vi "user_config.vi"(11 "ClusterIn":T2={"Simulation?"=FALSE, "ChanConfigs"=[], "Test Config"={"HoleDiam"=1.4, "MeanLineDiam"=5.0, "IncF"=0.2, "ElastMod"=207.0, "PoissonMod"=0.3, "RosType"=enum."Tipo A", "Método de análise"=enum."Simplificado 2008", "Pfinal"=0.3, "AStop"=TRUE}, "Directory"=path "", "TestName"="", "RawFile"=refnum, "InfoFile"=refnum, "DataFile"=refnum, "task"="", "qRecord"=refnum, "qProcess"=refnum, "feed"=enum."Manual"} {"ChanConfigs"."GF" min=0.1 max=10.0; "ChanConfigs"."Canal" min=1 max=8}) -> (3 "ClusterOut":T2={"Simulation?"=FALSE, "ChanConfigs"=[], "Test Config"={"HoleDiam"=1.4, "MeanLineDiam"=5.0, "IncF"=0.2, "ElastMod"=207.0, "PoissonMod"=0.3, "RosType"=enum."Tipo A", "Método de análise"=enum."Simplificado 2008", "Pfinal"=0.3, "AStop"=TRUE}, "Directory"=path "", "TestName"="", "RawFile"=refnum, "InfoFile"=refnum, "DataFile"=refnum, "task"="", "qRecord"=refnum, "qProcess"=refnum, "feed"=enum."Manual"} {"ChanConfigs"."GF" min=0.1 max=10.0; "ChanConfigs"."Canal" min=1 max=8})   [LabVIEW 2016]
uses:
  Channel_config.ctl
  MainFGV/cluster_main_FGV.ctl
  test_config.ctl
  feedType.ctl
panel:
  in  "feed":T1 caption="Tipo de avanço"
  in  "ChanConfig":T3[](array[typedef])=[{"Canal"=1, "GF"=2.0, "SC"=FALSE}, {"Canal"=2, "GF"=2.0, "SC"=FALSE}, {"Canal"=3, "GF"=2.0, "SC"=FALSE}] {"GF" min=0.1 max=10.0; "Canal" min=1 max=8}
  in  "Parar auto.":bool=TRUE
  in  "Pf":dbl=1.0 caption="Profundidade final [mm]"
  in  "TR":enum16{"Tipo A", "Tipo B", "Tipo C"}(ring) caption="Tipo de roseta utilizada"
  in  "ni":dbl=0.3 caption="Módulo de Poisson"
  in  "E":dbl=207.0 caption="Módulo de elasticidade [GPa]"
  in  "IF":dbl=0.05 caption="Incremento de furação [mm]"
  in  "Dlm":dbl=5.13 caption="Diâmetro da linha média [mm]"
  in  "Df":dbl=1.4 caption="Diâmetro do furo [mm]"
  in  "Pronto":bool
  # "CONFIGURAÇÃO DO ENSAIO DE TENSÃO RESIDUAL"
  # "Informações essenciais para execução do ensaio"
  # "Sensor 1"
  # "Sensor 2"
  # "Sensor 3"
  # "Informações que serão usadas no processamento (podem ser informadas depois)"
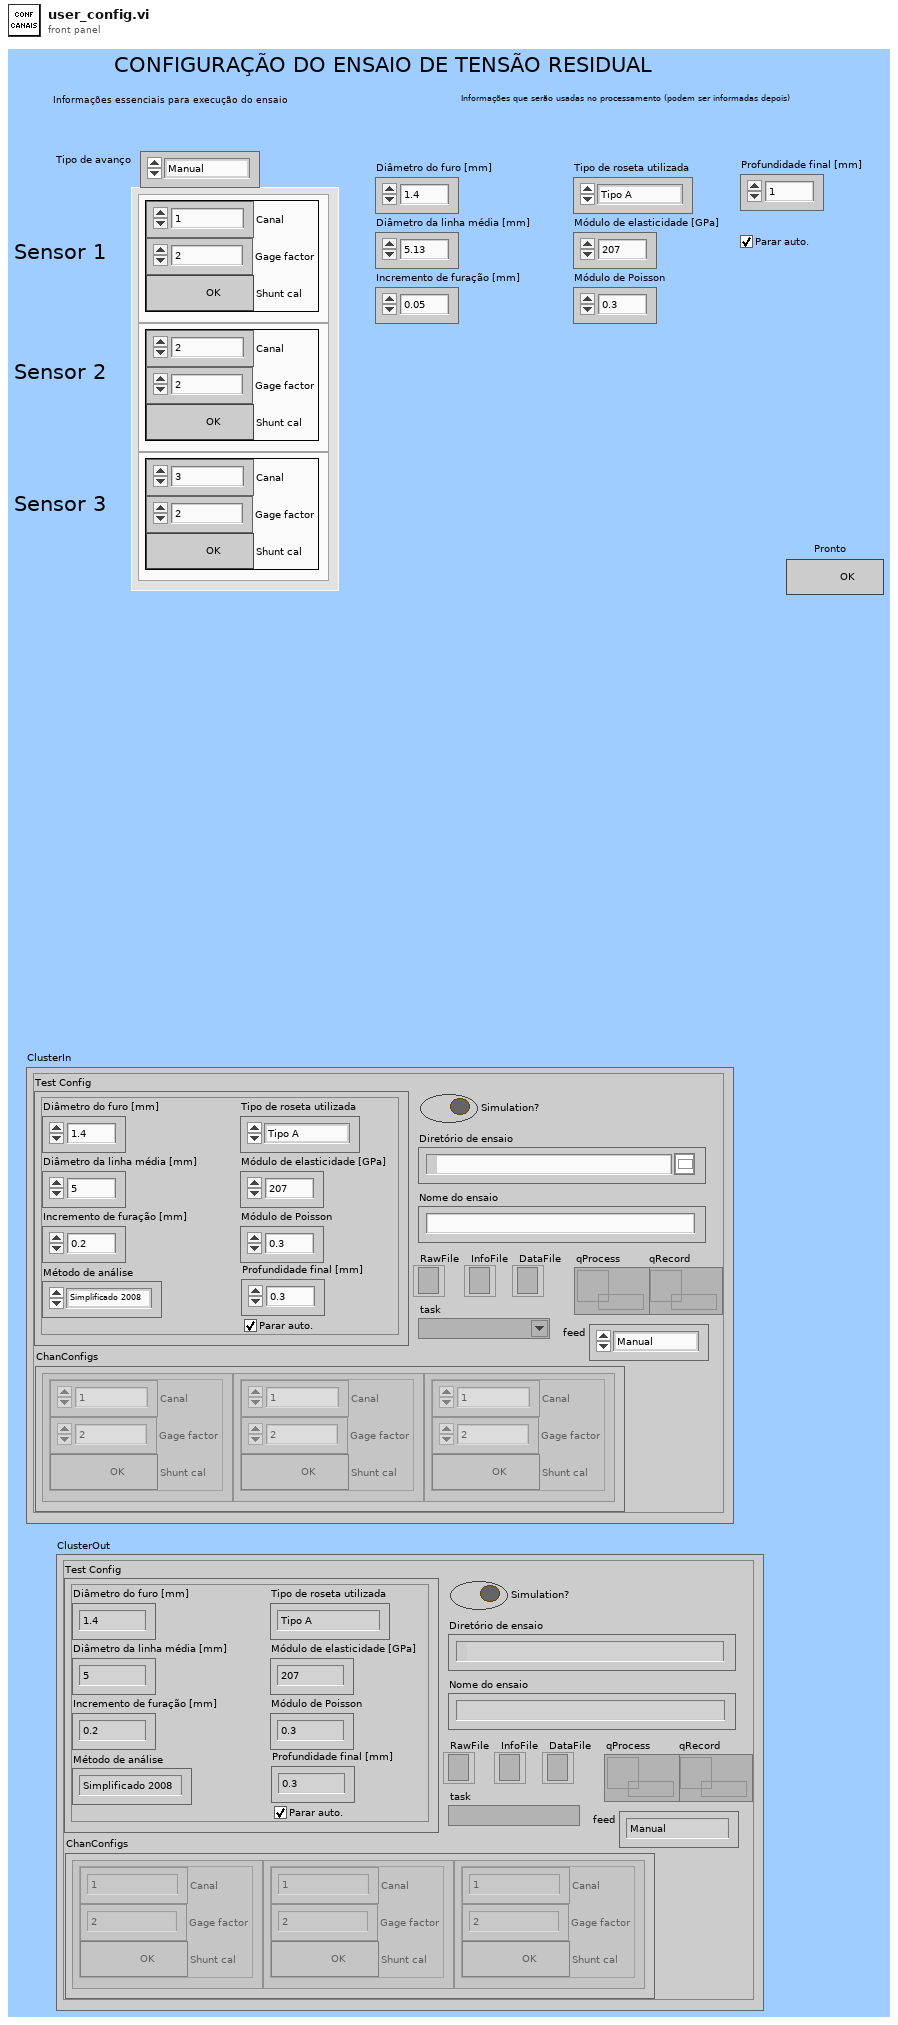
[diagram p1: front panel]
types:
  T1 = typedef "feedType.ctl" = enum16{"Manual", "Automático"}
  T2 = typedef "cluster_main_FGV.ctl" = cluster{"Simulation?":bool, "ChanConfigs":T3[], "Test Config":T4, "Directory":path, "TestName":string, "RawFile":refnum<file>, "InfoFile":refnum<file>, "DataFile":refnum<file>, "task":refnum<k21>, "qRecord":refnum<queue>, "qProcess":refnum<queue>, "feed":T1}
  T3 = typedef "Channel_config.ctl" = cluster{"Canal":i32, "GF":dbl, "SC":bool}
  T4 = typedef "test_config.ctl" = cluster{"HoleDiam":dbl, "MeanLineDiam":dbl, "IncF":dbl, "ElastMod":dbl, "PoissonMod":dbl, "RosType":enum16{"Tipo A", "Tipo B", "Tipo C"}, "Método de análise":enum16{"Não uniforme 2013", "Simplificado 2013", "Simplificado 2008"}, "Pfinal":dbl, "AStop":bool}
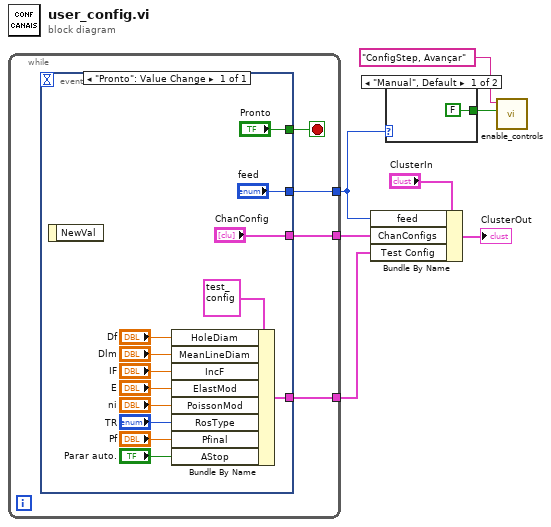
[diagram p0: block diagram]
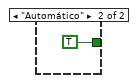
[diagram p2: hidden frame]
diagram:
  n1 = while {
    tunnel: [w10] -> w6
    tunnel: [w9] -> w5
    tunnel: [w8] -> w3
    stop <- w11 stop-if-true
    n2 = event shown="[0] \"Pronto\": Value Change" {
      selector: _ -> [_]
      dyn-events: _ -> [_]
      timeout: _ -> [_]
      tunnel: ["Pronto"] -> w11
      tunnel: [w17] -> w10
      tunnel: ["ChanConfig"] -> w9
      tunnel: ["feed"] -> w8
      event "Pronto": Value Change {
        n3 = event-data() -> ()  [unwired: 1 in, 1 out]
        n4 = Bundle By Name(cluster=T4 {"HoleDiam"=1.4, "MeanLineDiam"=5.0, "IncF"=0.2, "ElastMod"=207.0, "PoissonMod"=0.3, "RosType"=enum."Tipo A", "Método de análise"=enum."Simplificado 2008", "Pfinal"=0.3, "AStop"=TRUE} ("Test Config"), "HoleDiam"="Df", "MeanLineDiam"="Dlm", "IncF"="IF", "ElastMod"="E", "PoissonMod"="ni", "RosType"="TR", "Pfinal"="Pf", "AStop"="Parar auto.") -> (w17:T4)
      }
    }
  }
  n5 = Bundle By Name(cluster="ClusterIn", "feed"=w3, "ChanConfigs"=w5, "Test Config"=w6) -> (→"ClusterOut":T2)
  n6 = case shown="\"Manual\", Default" w3 {
    tunnel: [FALSE ("Enable?") TRUE ("Enable?")] -> w1
    frame "Manual", Default {
    }
    frame "Automático" {
    }
  }
  n7 = call "enable_controls.vi"("Enable?"=w1, "Controls Label"="ConfigStep, Avançar" ("name (unnamed)")) -> ()  [unwired: 9 in, 1 out]
